vi "仿真实验1-正弦非整周期采样直流分量.vi"() -> ()   [LabVIEW 2017]
uses:
  <vilib>/Analysis/4window.llb/windowTd.ctl
  <vilib>/measure/mascope.llb/Pulse Measurements 1 chan.vi
  <vilib>/measure/matone.llb/Extract Single Tone Information 1 Chan.vi
  <vilib>/measure/NI_MAPro.lvlib
  <vilib>/Analysis/NI_AALPro.lvlib
panel:
  in  "formula":string="sin(w*t)*sin(2*pi(1)*t)" caption="公式"
  out "FFTHanning窗校正":dbl
  out "FFT矩形窗校正":dbl
  out "三点法":dbl
  out "峰值多周期":dbl
  out "直流分量":dbl
  in  "幅值":dbl
  out "脉冲测量法":dbl
  out "过零插值":dbl
  out "过零多周期":dbl
  in  "频率":dbl
  out "提取单频信息":dbl caption="检测到的频率" format="%.6p"
  out "FFT":dbl
  in  "采样信息":cluster{"Fs":dbl, "#s":dbl}={"Fs"=1000.0, "#s"=1000.0}
  out "过零比较法":dbl
  out "波形图":waveform(dbl)(graph)
  # "仿真信号参数设置"
  # "频率测量结果"
  # "时域算法"
  # "频域算法"
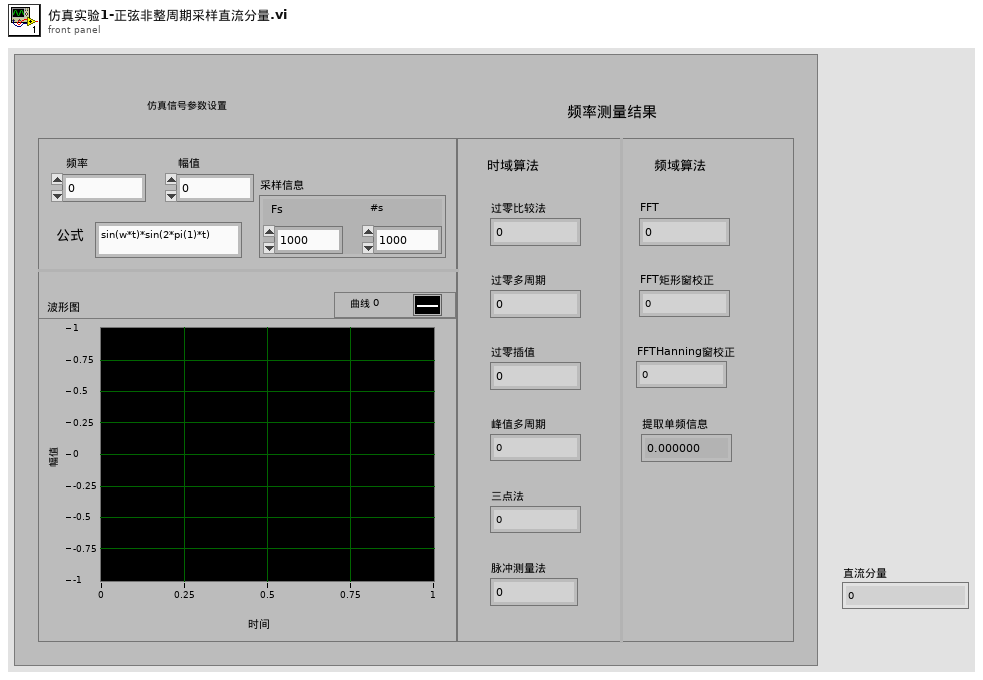
[diagram p1: front panel]
types:
  T1 = typedef "NI_AALPro.lvlib/windowTd.ctl" = u32
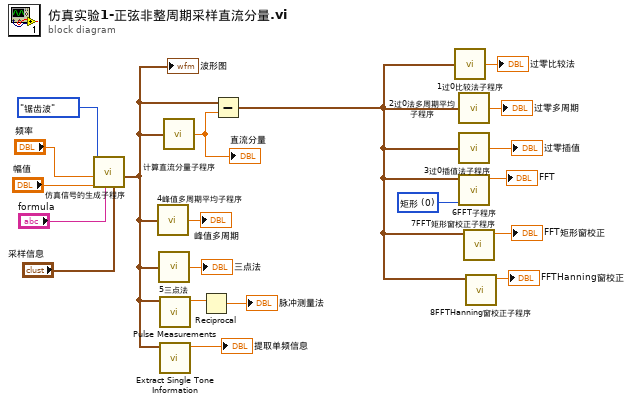
[diagram p0: block diagram]
diagram:
  w3 = T1 0 items=["矩形"=0, "Hanning"=1, "Hamming"=2, "Blackman-Harris"=3, "Exact Blackman"=4, "Blackman"=5, "Flat Top"=6, "4阶Blackman-Harris "=7, "7阶Blackman-Harris"=8, "Low Sidelobe"=9, "Blackman Nuttall"=11, "三角"=30, "Bartlett-Hanning"=31, "Bohman"=32, "Parzen"=33, "Welch"=34, "Kaiser"=60, "Dolph-Chebyshev"=61, "高斯"=62] ("window")
  n1 = call "仿真信号的生成子程序.vi"("sampling info"="采样信息", "formula"="formula", "幅值"="幅值", "频率"="频率", "波形选择"=enum16{"正弦波", "锯齿波", "三角波", "方波", "公式波"}."锯齿波") -> ("波形图"=w8:waveform(dbl))  [unwired: 6 in]
  "波形图" <- w8
  n2 = call "4峰值多周期平均子程序.vi"("波形"=w8) -> ("f"=→"峰值多周期":dbl)
  n3 = call "5三点法.vi"("波形"=w8) -> ("f"=→"三点法":dbl)
  n4 = call-poly <vilib>:"Pulse Measurements.vi"("signal in"=w8) -> ("period"=w13:dbl)  [unwired: 6 in, 4 out]
  n5 = call-poly <vilib>:"Extract Single Tone Information.vi"("time signal in"=w8) -> ("detected frequency"=→"提取单频信息":dbl)  [unwired: 5 in, 5 out]
  n6 = call "计算直流分量子程序.vi"("波形"=w8) -> ("直流分量"=w10:dbl)
  "直流分量" <- w10
  n7 = Reciprocal(x=w13) -> (1/x=→"脉冲测量法":dbl)
  n8 = Subtract(x=w8, y=w10) -> (x-y=w5:waveform(dbl))
  n9 = call "1过0比较法子程序.vi"("波形"=w5) -> ("f"=→"过零比较法":dbl)
  n10 = call "2过0法多周期平均子程序.vi"("波形"=w5) -> ("f"=→"过零多周期":dbl)
  n11 = call "3过0插值法子程序.vi"("波形"=w5) -> ("f"=→"过零插值":dbl)
  n12 = call "6FFT子程序.vi"("window"=w3, "time signal"=w5) -> ("频率"=→"FFT":dbl)  [unwired: 2 in, 3 out]
  n13 = call "7FFT矩形窗校正子程序.vi"("time signal"=w5) -> ("频率"=→"FFT矩形窗校正":dbl)  [unwired: 4 in, 2 out]
  n14 = call "8FFTHanning窗校正子程序.vi"("time signal"=w5) -> ("频率"=→"FFTHanning窗校正":dbl)  [unwired: 4 in, 2 out]
